vi "RawRT_Capture.vi"(5 "A/D bits":i16=8, 6 "Raw data":i16[][](array[numeric]), 7 "File Name In":string, 8 "Add Text":string="_raw", 9 "DigCard":i16, 10 "header":string, 11 "Iter":i16) -> ()   [LabVIEW 2022 SP3]
uses:
  ScanningControl/Motion Controllers/-MotionRoutines/MotionGlobals.vi
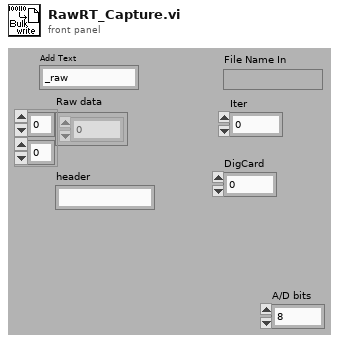
[diagram p1: front panel]
types:
  T1 = enum16{"open", "replace", "create", "open or create", "replace or create", "replace or create with confirmation"}
  T2 = enum16{"big-endian, network order", "native, host order", "little-endian"}
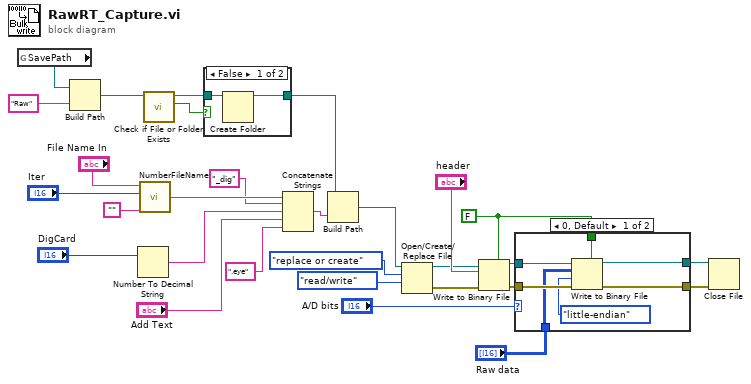
[diagram p0: block diagram]
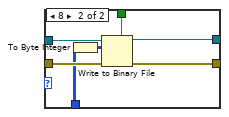
[diagram p3: hidden frame]
diagram:
  w13 = FALSE ("prepend array or string size? (T)")
  n1 = global read "MotionGlobals.vi" "SavePath"() -> (w8:path)
  n2 = Build Path(base path=w8, name or relative path="Raw") -> (appended path=w4:path)
  n3 = Number To Decimal String(number="DigCard") -> (decimal integer string=w21:string)  [unwired: 1 in]
  n4 = call "NumberFileName.vi"("String"="", "File number"="Iter", "file name"="File Name In") -> ("Numbered File"=w23:string)  [unwired: 1 in]
  n5 = call <vilib>:"Check if File or Folder Exists.vi"("path"=w4) -> ("file or folder exists?"=w3:bool, "dup path"=w1:path)  [unwired: 8 in, 1 out]
  n6 = case shown="False" w3 {
    tunnel: [w30 w32] -> w2
    tunnel: w1 -> [w31 w32]
    frame False {
      n7 = Create Folder(path (use dialog)=w31) -> (created path=w30:path)  [unwired: 2 in, 2 out]
    }
    frame True {
    }
  }
  n8 = Concatenate Strings(w23, "_dig", w21, "Add Text", ".eye") -> (w29:string)
  n9 = Build Path(base path=w2, name or relative path=w29) -> (appended path=w26:path)
  n10 = Open/Create/Replace File(file path (use dialog)=w26, operation (0:open)=T1."replace or create", access (0:read/write)=enum16{"read/write", "read-only", "write-only"}."read/write") -> (refnum out=w18:refnum<file>, error out=w17:errorcluster)  [unwired: 1 in, 3 out]
  n11 = Write to Binary File(file (use dialog)=w18, data="header", error in=w17, 5:w13) -> (refnum out=w16:refnum<file>, error out=w15:errorcluster)  [unwired: 2 in, 1 out]
  n12 = case shown="0, Default" "A/D bits" {
    tunnel: w16 -> [w39 w46]
    tunnel: w15 -> [w38 w45]
    tunnel: "Raw data" -> [w34 w44]
    tunnel: w13 -> [w37 w43]
    tunnel: [w36 w42] -> w12
    tunnel: [w35 w41] -> w11
    frame 0, Default {
      n13 = Write to Binary File(file (use dialog)=w39, data=w34, error in=w38, 5:w37, 9:T2."little-endian" ("byte order (0:big-endian, network order)")) -> (refnum out=w36:refnum<file>, error out=w35:errorcluster)  [unwired: 1 in, 1 out]
    }
    frame 8 {
      n14 = To Byte Integer(number=w44) -> (8bit integer=w40:i8[][])
      n15 = Write to Binary File(file (use dialog)=w46, data=w40, error in=w45, 5:w43) -> (refnum out=w42:refnum<file>, error out=w41:errorcluster)  [unwired: 2 in, 1 out]
    }
  }
  n16 = Close File(refnum=w12, error in=w11) -> ()  [unwired: 2 out]
